vi "PI Convert Limits Cluster.vi"(5 "Conversion":enum16{"Cluster - HTML", "HTML - Cluster"}(ring), 7 "PI Key Array In":T6, 8 "PI Cluster In":T1) -> (1 "PI Cluster Out":T1, 2 "PI HTML Out":string)   [LabVIEW 2011]
uses:
  Addons/internet/utils/keyedarr.llb/Keyed Array.ctl
  TypeDefs/PI Test Parameters.ctl
  TypeDefs/PI Measurement Cluster.ctl
  TypeDefs/PI Limit Parameters.ctl
  TypeDefs/PI Limit Definition.ctl
  TypeDefs/PI Limit Comparison.ctl
  Addons/internet/utils/strutil.llb/Case Matching.ctl
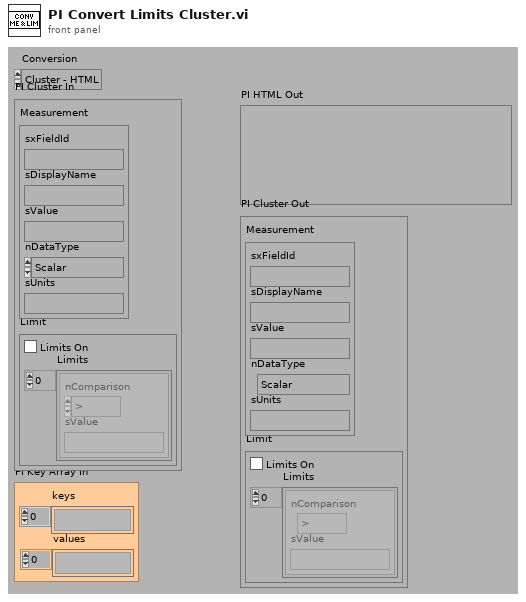
[diagram p1: front panel]
types:
  T1 = typedef "PI Test Parameters.ctl" = cluster{"Measurement":T2, "Limit":T3}
  T2 = typedef "PI Measurement Cluster.ctl" = cluster{"sxFieldId":string, "sValue":string, "nDataType":enum16{"Scalar", "Enumeration"}, "sUnits":string, "sDisplayName":string}
  T3 = typedef "PI Limit Parameters.ctl" = cluster{"Limits On":bool, "Limits":T4[]}
  T4 = typedef "PI Limit Definition.ctl" = cluster{"nComparison":T5, "sValue":string}
  T5 = typedef "PI Limit Comparison.ctl" = enum16{">", ">=", "<", "<=", "<>", "="}
  T6 = typedef "Keyed Array.ctl" = cluster{"keys":string[], "values":string[]}
  T7 = typedef "Case Matching.ctl" = enum16{"a != A", "a == A", "system"}
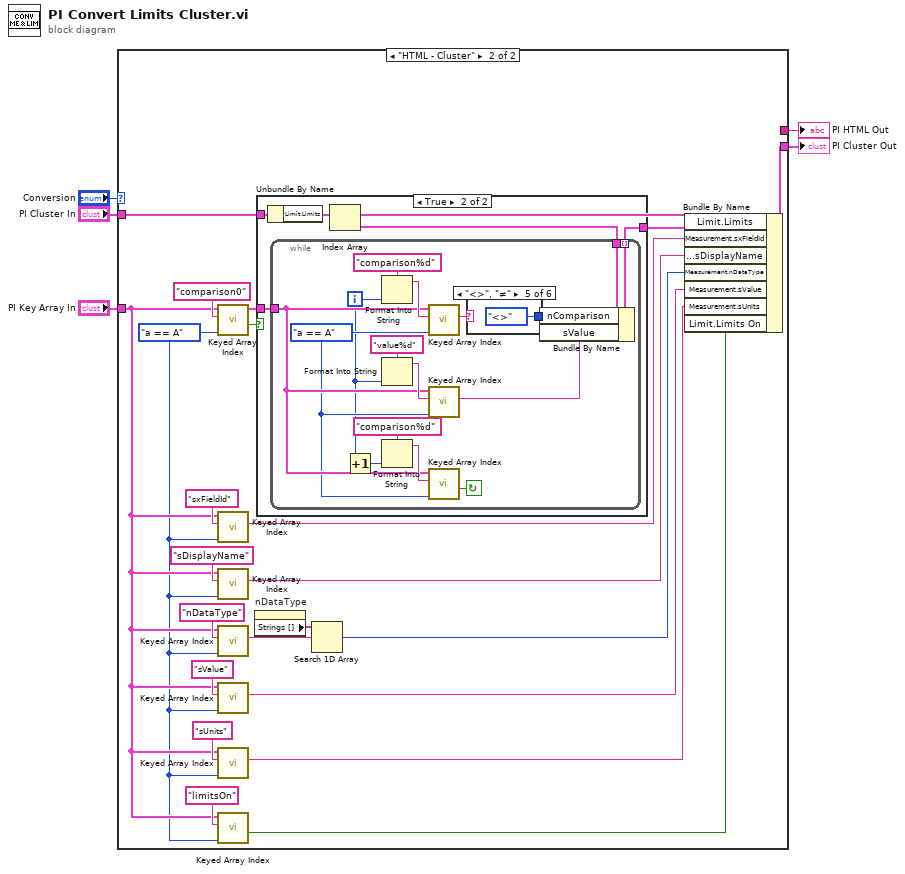
[diagram p0: block diagram]
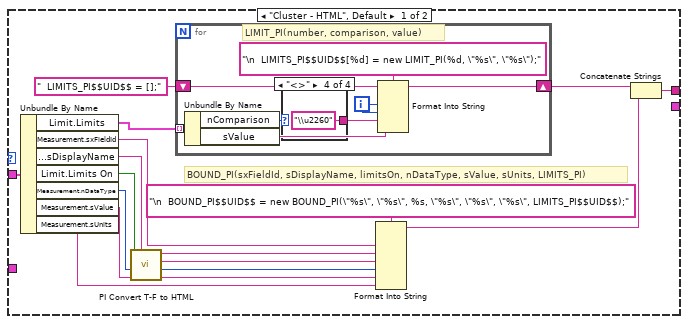
[diagram p2: hidden frame]
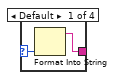
[diagram p3: hidden frame]
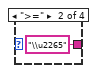
[diagram p4: hidden frame]
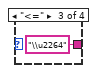
[diagram p5: hidden frame]
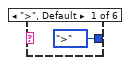
[diagram p7: hidden frame]
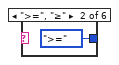
[diagram p8: hidden frame]
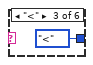
[diagram p9: hidden frame]
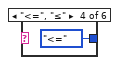
[diagram p10: hidden frame]
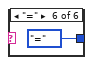
[diagram p11: hidden frame]
diagram:
  n1 = case shown="\"HTML - Cluster\"" "Conversion" {
    tunnel: "PI Cluster In" -> [w14 w47]
    tunnel: "PI Key Array In" -> [_ w35]
    tunnel: [w18 _] -> w2
    tunnel: [_ w48] -> w1
    frame "Cluster - HTML", Default {
      # "BOUND_PI(sxFieldId, sDisplayName, limitsOn, nDataType, sValue, sUnits, LIMITS_PI)"
      n2 = Unbundle By Name(w14) -> ("Limit.Limits"=w13:T4[], "Measurement.sxFieldId"=w12:string, "Measurement.sDisplayName"=w6:string, "Limit.Limits On"=w7:bool, "Measurement.nDataType"=w11:enum16{"Scalar", "Enumeration"}, "Measurement.sValue"=w10:string, "Measurement.sUnits"=w9:string)
      n3 = call "PI Convert T-F to HTML.vi"("(T/F)"=w7) -> ("HTML (true/false)"=w8:string)  [unwired: 10 out]
      n4 = for {
        tunnel: w13 -> [w27] mode=indexing
        shift-right: [w26] -> w17
        shift-left: "  LIMITS_PI$$UID$$ = [];" ("format string") -> [w22]
        i -> [w23]
        # "LIMIT_PI(number, comparison, value)"
        n5 = Unbundle By Name(w27) -> ("nComparison"=w21:T5, "sValue"=w24:string)
        n6 = case shown="\"<>\"" w21 {
          selector: w21 -> [w29 _ _ _]
          tunnel: [w28 "\\u2265" "\\u2264" "\\u2260"] -> w20
          frame Default {
            n7 = Format Into String(w29) -> (resulting string=w28:string)  [unwired: 3 in, 1 out]
          }
          frame ">=" {
          }
          frame "<=" {
          }
          frame "<>" {
          }
        }
        n8 = Format Into String(format string="\n  LIMITS_PI$$UID$$[%d] = new LIMIT_PI(%d, \"%s\", \"%s\");", initial string=w22, w23, w23, w20, w24) -> (resulting string=w26:string)  [unwired: 1 in, 1 out]
      }
      n9 = Format Into String(format string="\n  BOUND_PI$$UID$$ = new BOUND_PI(\"%s\", \"%s\", %s, \"%s\", \"%s\", \"%s\", LIMITS_PI$$UID$$);", w12, w6, w8, w11, w10, w9) -> (resulting string=w15:string)  [unwired: 2 in, 1 out]
      n10 = Concatenate Strings(w17, w15) -> (w18:string)
    }
    frame "HTML - Cluster" {
      w34 = Case_Matching."a == A" ("case matching (sensitive)")
      n11 = call "Keyed Array Index.vi"("case matching (sensitive)"=w34, "key"="comparison0", "array in"=w35) -> ("valid key"=w52:bool, "duplicate array"=w54:T6)  [unwired: 1 in, 2 out]
      n12 = call "Keyed Array Index.vi"("case matching (sensitive)"=w34, "key"="sxFieldId", "array in"=w35) -> ("value"=w50:string)  [unwired: 1 in, 3 out]
      n13 = call "Keyed Array Index.vi"("case matching (sensitive)"=w34, "key"="sDisplayName", "array in"=w35) -> ("value"=w33:string)  [unwired: 1 in, 3 out]
      n14 = call "Keyed Array Index.vi"("case matching (sensitive)"=w34, "key"="nDataType", "array in"=w35) -> ("value"=w45:string)  [unwired: 1 in, 3 out]
      n15 = call "Keyed Array Index.vi"("case matching (sensitive)"=w34, "key"="sValue", "array in"=w35) -> ("value"=w42:string)  [unwired: 1 in, 3 out]
      n16 = call "Keyed Array Index.vi"("case matching (sensitive)"=w34, "key"="sUnits", "array in"=w35) -> ("value"=w40:string)  [unwired: 1 in, 3 out]
      n17 = call "Keyed Array Index.vi"("case matching (sensitive)"=w34, "key"="limitsOn", "array in"=w35) -> ("valid key"=w38:bool)  [unwired: 1 in, 3 out]
      n18 = property on="nDataType" class="Enum (strict)"() -> ("Strings []"=w46:string[])  [unwired: 2 in, 2 out]
      n19 = case shown="True" w52 {
        tunnel: w47 -> [_ w57]
        tunnel: w54 -> [_ w59]
        tunnel: [_ w55] -> w49
        frame False {
        }
        frame True {
          n20 = Unbundle By Name(w57) -> ("Limit.Limits"=w56:T4[])
          n21 = Index Array(array=w56) -> (element=w58:T4)  [unwired: 1 in]
          n22 = while {
            tunnel: w58 -> [w75]
            tunnel: [w74] -> w55 mode=indexing
            tunnel: w59 -> [w65]
            i -> [w60]
            stop <- w66 continue-if-true
            w64 = Case_Matching."a == A" ("case matching (sensitive)")
            n23 = Increment(x=w60) -> (x+1=w67:i32)
            n24 = Format Into String(format string="comparison%d", w60) -> (resulting string=w73:string)  [unwired: 2 in, 1 out]
            n25 = Format Into String(format string="value%d", w60) -> (resulting string=w70:string)  [unwired: 2 in, 1 out]
            n26 = Format Into String(format string="comparison%d", w67) -> (resulting string=w69:string)  [unwired: 2 in, 1 out]
            n27 = call "Keyed Array Index.vi"("case matching (sensitive)"=w64, "key"=w73, "array in"=w65) -> ("value"=w63:string)  [unwired: 1 in, 3 out]
            n28 = call "Keyed Array Index.vi"("case matching (sensitive)"=w64, "key"=w70, "array in"=w65) -> ("value"=w61:string)  [unwired: 1 in, 3 out]
            n29 = call "Keyed Array Index.vi"("case matching (sensitive)"=w64, "key"=w69, "array in"=w65) -> ("valid key"=w66:bool)  [unwired: 1 in, 3 out]
            n30 = case shown="\"<>\", \"≠\"" w63 {
              tunnel: [PI_Limit_Comparison.">" ("Comparison") PI_Limit_Comparison.">=" ("Comparison") PI_Limit_Comparison."<" ("Comparison") PI_Limit_Comparison."<=" ("Comparison") PI_Limit_Comparison."<>" ("Comparison") PI_Limit_Comparison."=" ("Comparison")] -> w62
              frame ">", Default {
              }
              frame ">=", "≥" {
              }
              frame "<" {
              }
              frame "<=", "≤" {
              }
              frame "<>", "≠" {
              }
              frame "=" {
              }
            }
            n31 = Bundle By Name(cluster=w75, "nComparison"=w62, "sValue"=w61) -> (w74:T4)
          }
        }
      }
      n32 = Search 1D Array(1D array=w46, element=w45) -> (index of element=w44:i32)  [unwired: 1 out]
      n33 = Bundle By Name(cluster=w47, "Limit.Limits"=w49, "Measurement.sxFieldId"=w50, "Measurement.sDisplayName"=w33, "Measurement.nDataType"=w44, "Measurement.sValue"=w42, "Measurement.sUnits"=w40, "Limit.Limits On"=w38) -> (w48:T1)
    }
  }
  "PI HTML Out" <- w2
  "PI Cluster Out" <- w1
